vi "List All Case Frame Names.vi"(8 "error in (no error)":errorcluster, 11 "JKI SM in":refnum<class "JKI SM.lvclass">) -> (0 "error out":errorcluster, 1 "Event Structure Frame Names":string[](array[string]), 2 "Case Structure Frame Names":string[](array[string]), 3 "JKI SM out":refnum<class "JKI SM.lvclass">)   [LabVIEW 2020, in "JKI State Machine API.lvlib" / "JKI SM.lvclass"]
uses:
  JKI SM.lvclass
  JKI SM.lvclass/JKI SM.ctl
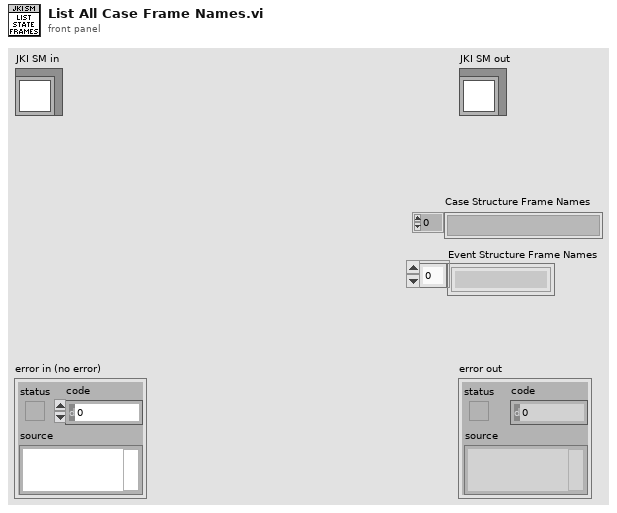
[diagram p1: front panel]
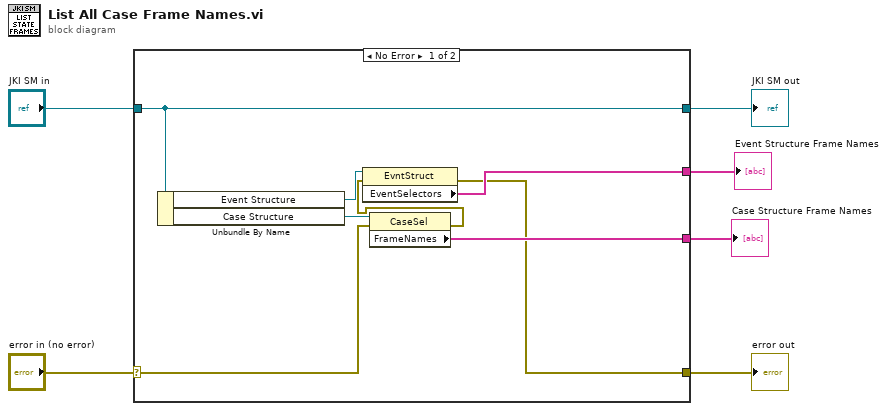
[diagram p0: block diagram]
diagram:
  n1 = case shown="No Error" "error in (no error)" {
    selector: "error in (no error)" -> [w12 w16]
    tunnel: [w7 w16] -> w5
    tunnel: [w14 w15] -> w3
    tunnel: "JKI SM in" -> [w14 w15]
    tunnel: [w11 _] -> w2
    tunnel: [w9 _] -> w1
    frame No Error {
      n2 = Unbundle By Name(w14) -> ("Event Structure"=w10:refnum<vi>, "Case Structure"=w13:refnum<vi>)
      n3 = property class="CaseSel"(reference=w13, error in=w12) -> (error out=w8:errorcluster, "FrameNames"=w11:string[])  [unwired: 1 out]
      n4 = property class="EvntStruct"(reference=w10, error in=w8) -> (error out=w7:errorcluster, "EventSelectors"=w9:string[])  [unwired: 1 out]
    }
    frame Error {
    }
  }
  "error out" <- w5
  "JKI SM out" <- w3
  "Case Structure Frame Names" <- w2
  "Event Structure Frame Names" <- w1
